vi "start.vi"(8 "error in (no error)":errorcluster, 11 "GenericToplevelComponent in":refnum<class "GenericToplevelComponent.lvclass">) -> (0 "error out":errorcluster, 3 "GenericToplevelComponent out":refnum<class "GenericToplevelComponent.lvclass">)   [LabVIEW 2010, in "GenericToplevelComponent.lvclass"]
uses:
  GenericToplevelComponent.lvclass
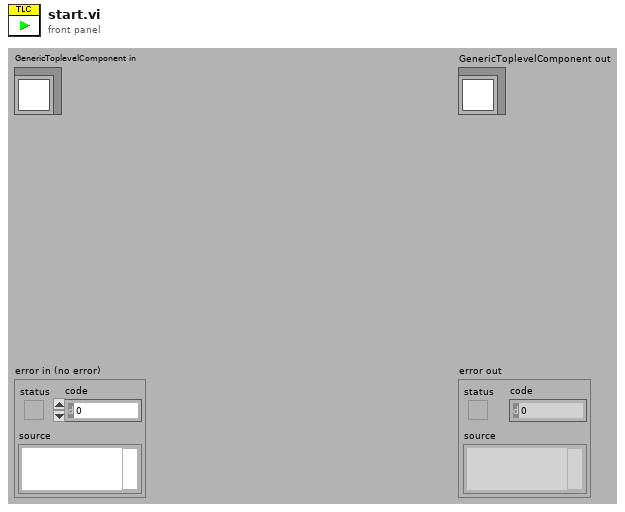
[diagram p1: front panel]
types:
  T1 = typedef "GenericToplevelComponent.lvclass/common_trigger_enum.ctl" = enum16{"NULL", "initialise", "terminate", "fetch command", "fetch data", "attach observer", "register as observer", "detach observer", "acknowledge", "start", "stop", "sweep started", "sweep finished", "experiment started", "experiment stopped"}
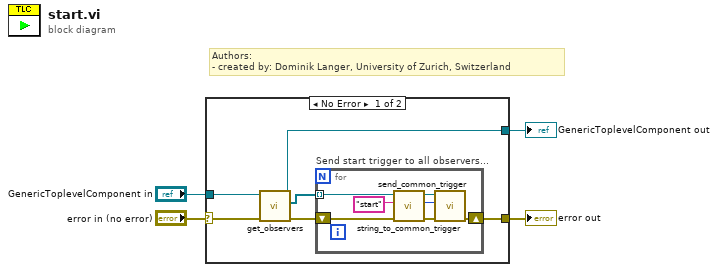
[diagram p0: block diagram]
diagram:
  # "Authors: \n- created by: Dominik Langer, University of Zurich, Switzerland"
  n1 = case shown="No Error" "error in (no error)" {
    selector: "error in (no error)" -> [w9 w19]
    tunnel: [w10 w19] -> w3
    tunnel: [w5 w18] -> w1
    tunnel: "GenericToplevelComponent in" -> [w6 w18]
    frame No Error {
      n2 = call-dynamic "get_observers.vi"("error in (no error)"=w9, "GenericToplevelComponent in"=w6) -> ("error out"=w8:errorcluster, "observers"=w7:refnum<class "GenericToplevelComponent.lvclass">[], "GenericToplevelComponent out"=w5:refnum<class "GenericToplevelComponent.lvclass">)  [unwired: 7 in]
      n3 = for "Send start trigger to all observers..." {
        shift-right: [w17] -> w10
        shift-left: w8 -> [w15]
        tunnel: w7 -> [w14] mode=indexing
        n4 = call-dynamic "string_to_common_trigger.vi"("error in (no error)"=w15, "trigger string"="start", "GenericToplevelComponent in"=w14) -> ("error out"=w12:errorcluster, "trigger"=w11:T1, "GenericToplevelComponent out"=w13:refnum<class "GenericToplevelComponent.lvclass">)  [unwired: 6 in]
        n5 = call-dynamic "send_common_trigger.vi"("error in (no error)"=w12, "trigger"=w11, "GenericToplevelComponent in"=w13) -> ("error out"=w17:errorcluster)  [unwired: 6 in, 2 out]
      }
    }
    frame Error {
    }
  }
  "error out" <- w3
  "GenericToplevelComponent out" <- w1
